vi "Read.vi"(11 "History Data Value in":refnum<class "Unix ns Data Value.lvclass">) -> (2 "Data":T1)   [LabVIEW 2020, in "VolatusHistorian.lvlib" / "Unix ns Data Value.lvclass"]
uses:
  Unix ns Data Value.lvclass
  History Data (unix ns).ctl
  Channel History (unix ns).ctl
  Unix ns Data Value.lvclass/Unix ns Data Value.ctl
  VolatusHistorian.lvlib
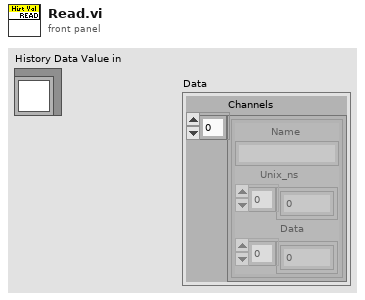
[diagram p1: front panel]
types:
  T1 = typedef "VolatusHistorian.lvlib/History Data (unix ns).ctl" = cluster{"Channels":T2[]}
  T2 = typedef "VolatusHistorian.lvlib/Channel History (unix ns).ctl" = cluster{"Name":string, "Unix_ns":i64[], "Data":dbl[]}
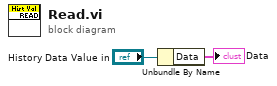
[diagram p0: block diagram]
diagram:
  n1 = Unbundle By Name("History Data Value in") -> ("Data"=→"Data":T1)
